vi "voltageMonitor.vi"(3 "Cell 1 voltage":dbl) -> (0 "Boolean":bool)   [LabVIEW 2014]
uses:
  <vilib>/imath/engines/lvmath2/RunTimeEngine/NodeEndStatement/NIMS_NodeEndStatement_Output.vi
  <instcachedir>/0/NIMS_NodeEndStatement_Output_53EC0D466D134D7ABD903AC30B43404B.lvgen/NIMS_NodeEndStatement_Output_53EC0D466D134D7ABD903AC30B43404B_011.vi
  <vilib>/imath/engines/lvmath2/RunTimeEngine/ErrorHandling/NIMS_Finalize Error.vi
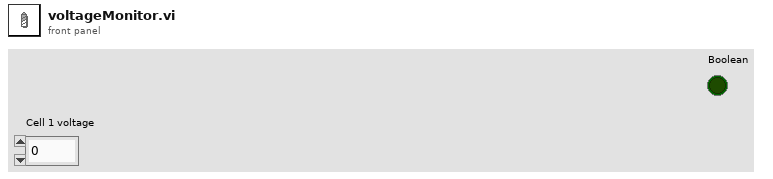
[diagram p1: front panel]
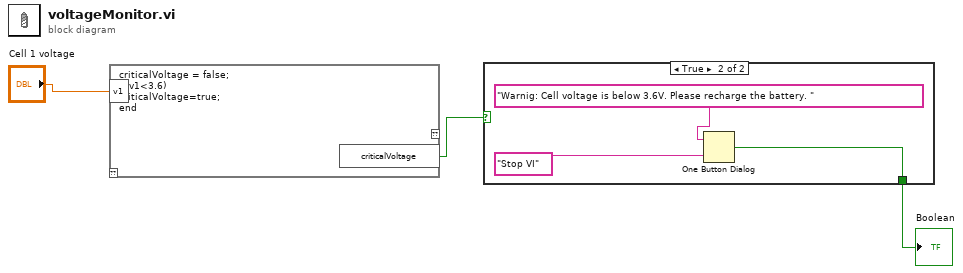
[diagram p0: block diagram]
diagram:
  n1 = mathscript code="criticalVoltage = false;\nif(v1<3.6)\ncriticalVoltage=true;\nend"("v1"="Cell 1 voltage") -> ("criticalVoltage"=w3:bool)  [unwired: 1 in, 1 out]
  n2 = case shown="True" w3 {
    selector: w3 -> [w4 _]
    tunnel: [w4 w5] -> w1
    frame False {
    }
    frame True {
      n3 = One Button Dialog(message="Warnig: Cell voltage is below 3.6V. Please recharge the battery. ", button name ("OK")="Stop VI") -> (true=w5:bool)
    }
  }
  "Boolean" <- w1
